vi "OpenCreate Dataset.vi"(4 "Datatype":variant, 5 "Chunk size":i32[](array[numeric]), 7 "deflate (5)":i32=5, 8 "error in (no error)":errorcluster, 10 "Dataset Path":string, 11 "HDF5 Ref":T1) -> (0 "error out":errorcluster, 2 "HDF5 Dataset Ref out":T1, 3 "HDF5 Ref out":T1)   [LabVIEW 2012]
doc: "Opens, creates, or replaces a dataset.\n\nHDF5 Ref: A file or group reference to the base location of the dataset\n\nDataset Path: The remainder of the path. This string may contain multiple subgroup elements separated by '/'. If the groups do not exist, they will be created. The final element of the path is the dataset name.\n\nDatatype and Dataspace: wire data to this input that matches the type and dimentionality of the dataset.\n\nUnlimited dataset: If true, a dataset extendable in all dimensions will be created.\n\nReplace Existing: if a dataset with the same name and path already exists, it will be replaced if this value is true. If ihe dataset exists and the value is false, an error will occur. \n\nChunk size: controls the block size in which space is allocated for unlimited datasets. The length of this array must match the rank of the data wired to Datatype and Dataspace. If unwired, it defaults to 1 in all dimensions."
uses:
  <vilib>/addons/_hdf5/library.llb/HDF5 Ref.ctl
  <vilib>/addons/_hdf5/property.llb/H5D_layout_t.ctl
panel:
  # "Copyright (c) 2005-2006 by Jason D. Sommerville                 \n\nThis program is free software; you can redistribute it and/or modify  it under the terms of the Common Public License Version 1.0 as  published by the Open Source Initiative.                          \n\nThis program is distributed in the hope that it will be useful, but WITHOUT ANY WARRANTY; without even the implied warranty of  MERCHANTABILITY or FITNESS FOR A PARTICULAR PURPOSE.  See the Common Public License for more details. \n\nYou should have received a copy of the Common Public License along with this program; if not, visit the OSI website at http://www.opensource.org/"
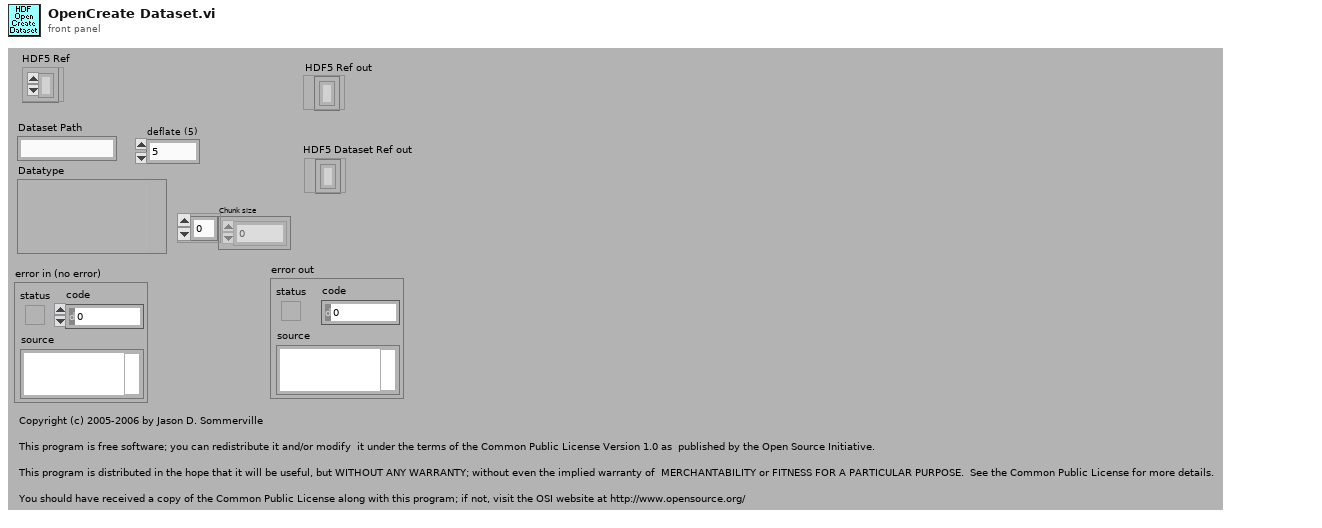
[diagram p1: front panel]
types:
  T1 = typedef "HDF5 Ref.ctl" = refnum<k1>
  T2 = enum32{"H5P_NO_CLASS_DEFAULT", "H5P_FILE_CREATE_DEFAULT", "H5P_FILE_ACCESS_DEFAULT", "H5P_DATASET_CREATE_DEFAULT", "H5P_DATASET_XFER_DEFAULT", "H5P_MOUNT_DEFAULT"}
  T3 = typedef "H5D_layout_t.ctl" = i32
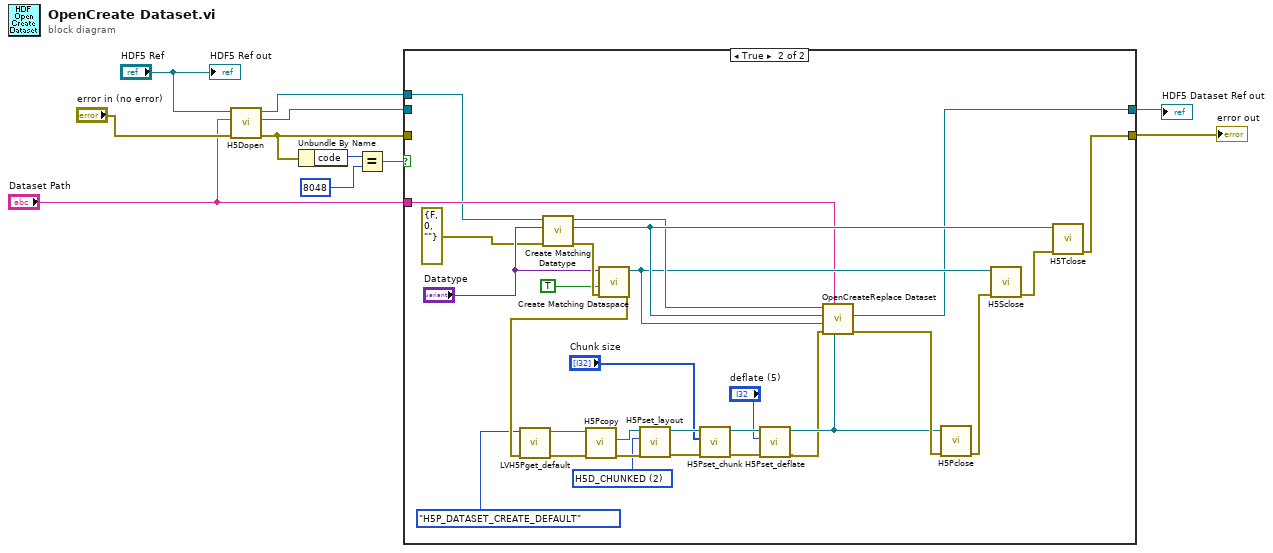
[diagram p0: block diagram]
diagram:
  n1 = call <vilib>:"H5Dopen.vi"("error in (no error)"="error in (no error)", "name"="Dataset Path", "HDF5 Ref"="HDF5 Ref") -> ("error out"=w3:errorcluster, "HDF5 Dataset Ref"=w4:T1, "HDF5 Ref out"=w2:T1)  [unwired: 4 in]
  n2 = Unbundle By Name(w3) -> ("code"=w7:i32)
  n3 = Equal?(x=w7, y=8048) -> (x = y?=w5:bool)
  n4 = case shown="True" w5 {
    tunnel: [w12 w37] -> w11
    tunnel: "Dataset Path" -> [_ w19]
    tunnel: w4 -> [w13 _]
    tunnel: [w13 w15] -> w1
    tunnel: w3 -> [w12 _]
    tunnel: w2 -> [_ w17]
    frame False {
    }
    frame True {
      w29 = T3 2 items=["H5D_LAYOUT_ERROR"=-1, "H5D_COMPACT"=0, "H5D_CONTIGUOUS"=1, "H5D_CHUNKED"=2] ("Layout")
      n5 = call <vilib>:"Create Matching Datatype.vi"("error in (no error)"=errorcluster {"status"=FALSE, "code"=0, "source"=""}, "Data"="Datatype", "HDF5 Ref"=w17) -> ("error out"=w40:errorcluster, "HDF5 Type Ref"=w42:T1, "HDF5 Ref out"=w39:T1)  [unwired: 4 in]
      n6 = call <vilib>:"Create Matching Dataspace.vi"("error in (no error)"=w40, "Max size unlimited (F)"=TRUE, "Data"="Datatype") -> ("error out"=w36:errorcluster, "HDF5 Dataspace Ref"=w38:T1)  [unwired: 5 in]
      n7 = call <vilib>:"LVH5Pget_default.vi"("error in (no error)"=w36, "Default Property List"=T2."H5P_DATASET_CREATE_DEFAULT") -> ("error out"=w35:errorcluster, "HDF5 Property List Ref"=w34:T1)  [unwired: 6 in]
      n8 = call <vilib>:"H5Pcopy.vi"("error in (no error)"=w35, "HDF5 Property Ref"=w34) -> ("error out"=w31:errorcluster, "HDF5 Property Ref Copy"=w30:T1)  [unwired: 5 in, 1 out]
      n9 = call <vilib>:"H5Pset_layout.vi"("error in (no error)"=w31, "Layout"=w29, "HDF5 Property Ref"=w30) -> ("error out"=w27:errorcluster, "HDF5 Ref out"=w28:T1)  [unwired: 5 in]
      n10 = call <vilib>:"H5Pset_chunk.vi"("error in (no error)"=w27, "Dimensions"="Chunk size", "HDF5 Property Ref"=w28) -> ("error out"=w23:errorcluster, "HDF5 Ref out"=w24:T1)  [unwired: 5 in]
      n11 = call <vilib>:"H5Pset_deflate.vi"("error in (no error)"=w23, "Level (5)"="deflate (5)", "HDF5 Property Ref"=w24) -> ("error out"=w21:errorcluster, "HDF5 Ref out"=w22:T1)  [unwired: 5 in]
      n12 = call <vilib>:"OpenCreateReplace Dataset.vi"("HDF5 Property List Ref"=w22, "Name"=w19, "error in (no error)"=w21, "HDF5 Dataspace Ref"=w38, "HDF5 Datatype Ref"=w42, "HDF5 Ref"=w39) -> ("error out"=w32:errorcluster, "HDF5 Dataset Ref"=w15:T1)  [unwired: 3 in, 1 out]
      n13 = call <vilib>:"H5Pclose.vi"("error in (no error)"=w32, "HDF5 Property Ref"=w22) -> ("error out"=w33:errorcluster)  [unwired: 7 in]
      n14 = call <vilib>:"H5Sclose.vi"("error in (no error)"=w33, "HDF5 Dataspace Ref"=w38) -> ("error out"=w41:errorcluster)  [unwired: 7 in]
      n15 = call <vilib>:"H5Tclose.vi"("error in (no error)"=w41, "HDF5 Datatype Ref"=w42) -> ("error out"=w37:errorcluster)  [unwired: 7 in]
    }
  }
  "error out" <- w11
  "HDF5 Dataset Ref out" <- w1
  "HDF5 Ref out" <- "HDF5 Ref"
